vi "Get Start End Angles.vi"(11 "Search":enum32{"Upper", "Lower"}(ring)) -> (2 "Start Angle (degrees)":dbl, 3 "End Angle (degrees)":dbl)   [LabVIEW 2015]
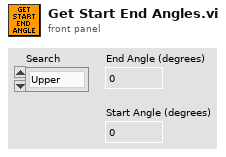
[diagram p1: front panel]
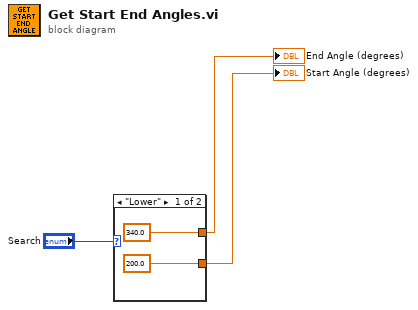
[diagram p0: block diagram]
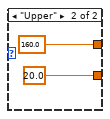
[diagram p2: hidden frame]
diagram:
  n1 = case shown="\"Lower\"" "Search" {
    tunnel: [200.0 ("Start Angle (degrees)") 20.0 ("Start Angle (degrees)")] -> w3
    tunnel: [340.0 ("End Angle (degrees)") 160.0 ("End Angle (degrees)")] -> w2
    frame "Lower" {
    }
    frame "Upper" {
    }
  }
  "Start Angle (degrees)" <- w3
  "End Angle (degrees)" <- w2
